vi "Seperated Exclusive Or.vi"(9 "q":bool, 10 "p":bool) -> (1 "only q":bool, 2 "only p":bool)   [LabVIEW 2019]
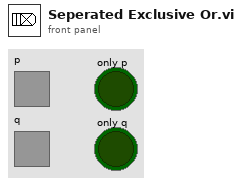
[diagram p1: front panel]
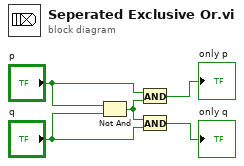
[diagram p0: block diagram]
diagram:
  n1 = Not And(1:"q", 2:"p") -> (0:w5:bool)
  n2 = And(x="p", y=w5) -> (x .and. y?=→"only p":bool)
  n3 = And(x=w5, y="q") -> (x .and. y?=→"only q":bool)
